vi "dvm Close.vi"(8 "error in (no error)":errorcluster, 11 "dvm session in":T1={"type"=enum."Disabled", "idn"="", "F5790"={"VISA"="", "Input"=enum."input 1", "Digital filter restart"=enum."medium", "hi resolution"=enum."off", "Digital filter mode"=enum."off", "ext guard"=FALSE}, "HP3458A"={"VISA"="", "ac method"=0, " resolution"=enum."6.5", "function"=0, "frequency source"=3, "auto range"=1, "manual range"=1.0}} {"HP3458A"."manual range" format="%_3g"; "HP3458A"."auto range" items=["OFF", "ON", "ONCE"]; "HP3458A"."frequency source" items=["AC + DC Current", "AC + DC Voltage", "AC Current", "AC Voltage"]; "HP3458A"."function" items=["DC Voltage", "AC Voltage", "AC + DC Voltage", "DC Current", "AC Current", "AC + DC Current", "2-Wire Resistance", "4-Wire Resistance", "Frequency", "Period", "Direct Sampling DC", "Direct Sampling AC", "Sub-Sampling DC", "Sub-Sampling AC"]; "HP3458A"."ac method" items=["Analog", "Random", "Synchronous"]}) -> (0 "error out":errorcluster, 3 "dvm session out":T1={"type"=enum."Disabled", "idn"="", "F5790"={"VISA"="", "Input"=enum."input 1", "Digital filter restart"=enum."medium", "hi resolution"=enum."off", "Digital filter mode"=enum."off", "ext guard"=FALSE}, "HP3458A"={"VISA"="", "ac method"=0, " resolution"=enum."6.5", "function"=0, "frequency source"=3, "auto range"=1, "manual range"=1.0}} {"HP3458A"."manual range" format="%_3g"; "HP3458A"."auto range" items=["OFF", "ON", "ONCE"]; "HP3458A"."frequency source" items=["AC + DC Current", "AC + DC Voltage", "AC Current", "AC Voltage"]; "HP3458A"."function" items=["DC Voltage", "AC Voltage", "AC + DC Voltage", "DC Current", "AC Current", "AC + DC Current", "2-Wire Resistance", "4-Wire Resistance", "Frequency", "Period", "Direct Sampling DC", "Direct Sampling AC", "Sub-Sampling DC", "Sub-Sampling AC"]; "HP3458A"."ac method" items=["Analog", "Random", "Synchronous"]})   [LabVIEW 2020]
doc: "Close auxiliary DVM."
uses:
  dvm session.ctl
  dvm type.ctl
  drivers/Fluke 5790A/top_level/F5790 session.ctl
  drivers/Agilent 3458A/top level/HP3458A Session.ctl
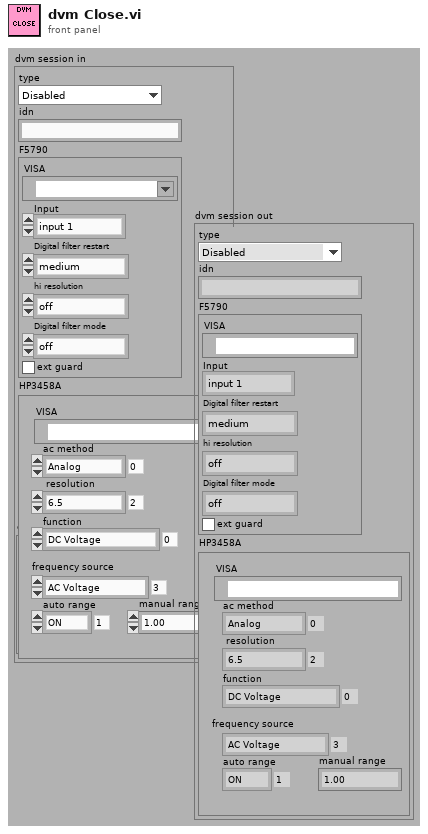
[diagram p1: front panel]
types:
  T1 = typedef "dvm session.ctl" = cluster{"type":T2, "idn":string, "F5790":T3, "HP3458A":T4}
  T2 = typedef "dvm type.ctl" = enum16{"Disabled", "Simulated", "Fluke 5790A", "Keysight 3458A"}
  T3 = typedef "F5790 session.ctl" = cluster{"VISA":refnum<visa-resource-name>, "Input":enum16{"input 1", "input 2", "wide-band"}, "Digital filter restart":enum16{"medium", "fine", "coarse"}, "hi resolution":enum16{"off", "on"}, "Digital filter mode":enum16{"off", "fast", "medium", "slow"}, "ext guard":bool}
  T4 = typedef "HP3458A Session.ctl" = cluster{"VISA":refnum<visa-resource-name>, "ac method":u16, " resolution":enum16{"4.5", "5.5", "6.5", "7.5", "8.5"}, "function":u16, "frequency source":u16, "auto range":u16, "manual range":dbl}
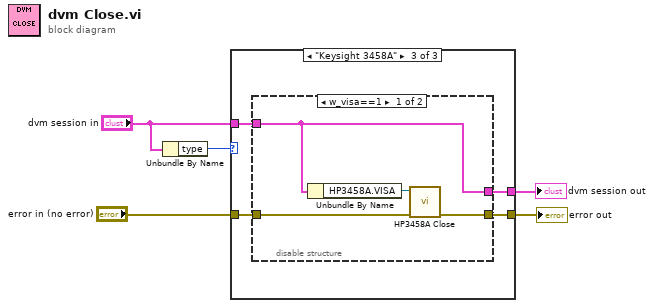
[diagram p0: block diagram]
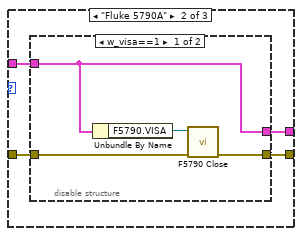
[diagram p3: hidden frame]
diagram:
  n1 = Unbundle By Name("dvm session in") -> ("type"=w5:T2)
  n2 = case shown="\"Keysight 3458A\"" w5 {
    tunnel: "dvm session in" -> [w6 w10 w20]
    tunnel: "error in (no error)" -> [w7 w11 w21]
    tunnel: [w7 w9 w19] -> w2
    tunnel: [w6 w8 w18] -> w1
    frame "Disabled", Default {
    }
    frame "Fluke 5790A" {
      n3 = disable-structure shown="w_visa==1" {
        disable-tunnel: w11 -> [w14 w17]
        disable-tunnel: w10 -> [w15 w16]
        disable-tunnel: [w12 w17] -> w9
        disable-tunnel: [w15 w16] -> w8
        frame condition #0 (active) {
          n4 = Unbundle By Name(w15) -> ("F5790.VISA"=w13:refnum<visa-resource-name>)
          n5 = call "F5790 Close.vi"("error in (no error)"=w14, "VISA in"=w13) -> ("error out"=w12:errorcluster)  [unwired: 9 in]
        }
        frame condition #1 {
        }
      }
    }
    frame "Keysight 3458A" {
      n6 = disable-structure shown="w_visa==1" {
        disable-tunnel: w21 -> [w24 w27]
        disable-tunnel: w20 -> [w25 w26]
        disable-tunnel: [w22 w27] -> w19
        disable-tunnel: [w25 w26] -> w18
        frame condition #0 (active) {
          n7 = Unbundle By Name(w25) -> ("HP3458A.VISA"=w23:refnum<visa-resource-name>)
          n8 = call "HP3458A Close.vi"("error in (no error)"=w24, "VISA in"=w23) -> ("error out"=w22:errorcluster)  [unwired: 9 in]
        }
        frame condition #1 {
        }
      }
    }
  }
  "error out" <- w2
  "dvm session out" <- w1
